vi "Variant to Storage Event.vi"(8 "error in (no error)":errorcluster, 10 "variant":variant, 11 "Storage in":refnum<class "Storage.lvclass">) -> (0 "error out":errorcluster, 2 "Event Registration Refnum":refnum<event-registration>, 3 "Storage out":refnum<class "Storage.lvclass">)   [LabVIEW 2015, in "AMS UI.lvlib" / "Storage.lvclass"]
uses:
  Storage.lvclass
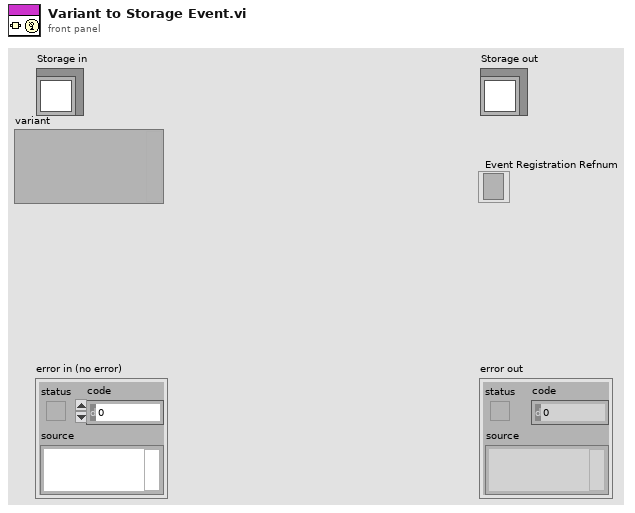
[diagram p1: front panel]
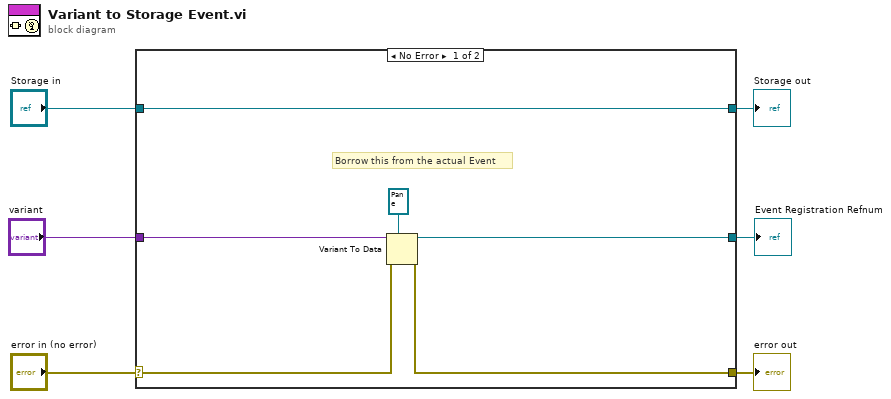
[diagram p0: block diagram]
diagram:
  n1 = case shown="No Error" "error in (no error)" {
    selector: "error in (no error)" -> [w11 w14]
    tunnel: [w10 w14] -> w5
    tunnel: [w12 w13] -> w3
    tunnel: "Storage in" -> [w12 w13]
    tunnel: "variant" -> [w9 _]
    tunnel: [w8 _] -> w1
    frame No Error {
      # "Borrow this from the actual Event"
      n2 = Variant To Data(error in=w11, type=refnum<event-registration> refnum ("event registration refnum"), Variant=w9) -> (data=w8:refnum<event-registration>, error out=w10:errorcluster)
    }
    frame Error {
    }
  }
  "error out" <- w5
  "Storage out" <- w3
  "Event Registration Refnum" <- w1
